vi "Read Key (Path).vi"(7 "section":string caption="Abschnitt", 8 "error in (no error)":errorcluster caption="Fehler (Eingang, kein Fehler)", 9 "default value":path caption="Standardwert", 10 "key":string caption="Schlüssel", 11 "refnum":T1 caption="RefNum") -> (0 "error out":errorcluster caption="Fehler (Ausgang)", 1 "value":path caption="Wert", 2 "found?":bool caption="Gefunden?", 3 "refnum out":T1 caption="RefNum (Ausgang)")   [LabVIEW 2009]
doc: "Liest einen Wert, der einem Schlüssel in einem angegebenen Abschnitt in der durch <B>Refnum</B> angegebenen Konfigurationsdatei zugeordnet ist. Wenn der Schlüssel nicht existiert, wird vom VI der Standardwert ausgegeben. Mit diesem polymorphen VI können folgende Wertetypen aus einem Schlüssel ausgelesen werden: boolesche Werte, numerische Werte mit doppelter Genauigkeit, vorzeichenbehaftete Integer-Werte, Pfade, Strings und vorzeichenlose Integer-Werte. Durch den Datentyp, der am Eingang <B>Index</B> anliegt, wird die zu verwendende Instanz des polymorphen VIs festgelegt."
uses:
  <vilib>/Utility/config.llb/Config Data RefNum.ctl
  <vilib>/Utility/config.llb/NI_LVConfig.lvlib
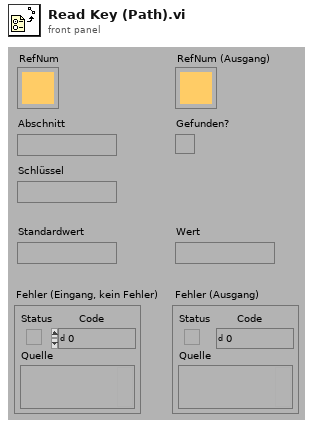
[diagram p1: front panel]
types:
  T1 = typedef "NI_LVConfig.lvlib/Config Data RefNum.ctl" = refnum<k1>
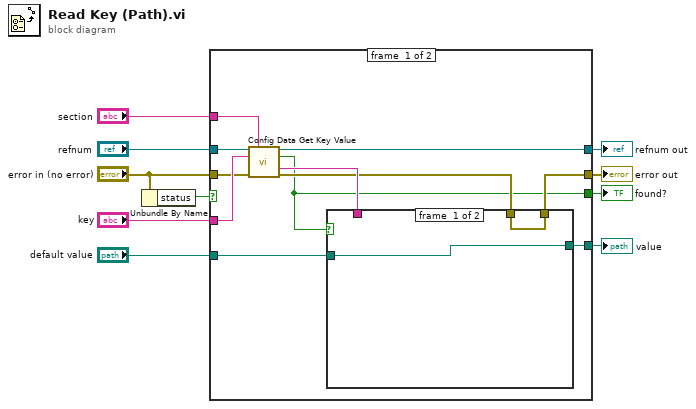
[diagram p0: block diagram]
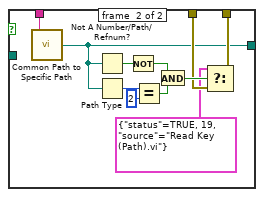
[diagram p2: hidden frame]
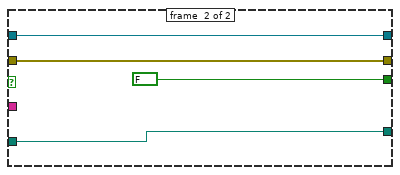
[diagram p3: hidden frame]
diagram:
  n1 = Unbundle By Name("error in (no error)") -> ("status"=w10:bool)
  n2 = case shown="False" w10 {
    tunnel: [w19 w37] -> w8
    tunnel: [w12 w38] -> w7
    tunnel: "refnum" -> [w16 w37]
    tunnel: "error in (no error)" -> [w17 w38]
    tunnel: "section" -> [w21 _]
    tunnel: "key" -> [w20 _]
    tunnel: [w11 FALSE ("section exists?")] -> w6
    tunnel: [w14 w36] -> w9
    tunnel: "default value" -> [w15 w36]
    frame #0 {
      n3 = call "Config Data Get Key Value.vi"("config data"=w16, "section"=w21, "key"=w20, "error in (no error)"=w17) -> ("config data out"=w19:T1, "key exists?"=w11:bool, "key value"=w18:string, "error out"=w13:errorcluster)  [unwired: 6 in, 2 out]
      n4 = case shown="True" w11 {
        tunnel: w18 -> [_ w34]
        tunnel: w15 -> [w23 _]
        tunnel: [w23 w24] -> w14
        tunnel: w13 -> [w22 w27]
        tunnel: [w22 w26] -> w12
        frame #0 {
        }
        frame #1 {
          n5 = call "Common Path to Specific Path.vi"("common path"=w34) -> ("specific path"=w24:path)  [unwired: 4 in]
          n6 = Not A Number/Path/Refnum?(number/path/refnum=w24) -> (NaN/Path/Refnum?=w31:bool)
          n7 = Path Type(1:w24) -> (0:w33:i16)
          n8 = Not(x=w31) -> (.not. x?=w30:bool)
          n9 = Equal?(x=w33, y=i16 2) -> (x = y?=w29:bool)
          n10 = And(x=w30, y=w29) -> (x .and. y?=w28:bool)
          n11 = Select(t=cluster{"status":bool, u16, "source":string} {"status"=TRUE, 19, "source"="Read Key (Path).vi"} ("f"), s=w28, f=w27) -> (s? t:f=w26:errorcluster)
        }
      }
    }
    frame #1 {
    }
  }
  "error out" <- w7
  "refnum out" <- w8
  "value" <- w9
  "found?" <- w6
